vi "Main3.vi"() -> ()   [LabVIEW 2014]
uses:
  TypeDefs/Errors.ctl
  TypeDefs/Data Info.ctl
  <vilib>/Utility/file.llb/Read From Spreadsheet File (string).vi
panel:
  out "Cluster 2":T2
  out "Day":T2={"Info 1"={"Last time in range?"=TRUE, "Date"="", "Start index"=0}, "Info 2"={"Last time in range?"=TRUE, "Date"="", "Start index"=0}, "Info 3"={"Last time in range?"=TRUE, "Date"="", "Start index"=0}, "Info 4"={"Last time in range?"=TRUE, "Date"="", "Start index"=0}, "info 5"={"Last time in range?"=TRUE, "Date"="", "Start index"=0}, "Info 6"={"Last time in range?"=TRUE, "Date"="", "Start index"=0}, "Info 7"={"Last time in range?"=TRUE, "Date"="", "Start index"=0}, "Info 8"={"Last time in range?"=TRUE, "Date"="", "Start index"=0}, "Info 9"={"Last time in range?"=TRUE, "Date"="", "Start index"=0}, "Info 10"={"Last time in range?"=TRUE, "Date"="", "Start index"=0}}
  in  "Cluster":T2
  out "Iteration":i32
  out "ADC Count":dbl[](array[numeric])
  out "# of rows":i32
  in  "Tab Control":T3(tab)
  out "Current (mA)":cluster{dbl[], dbl[]}(graph)
  out "XY Graph 10":cluster{dbl[], dbl[]}[](graph)
  out "Digital signals":cluster{dbl[], dbl[]}[](graph)
  out "Errors 1":T4
  out "Current (mA) 2":cluster{dbl[], dbl[]}(graph)
  out "XY Graph 11":cluster{dbl[], dbl[]}[](graph)
  out "Digital signals 3":cluster{dbl[], dbl[]}[](graph)
  out "Errors 2":T4
  out "Digital signals 2":cluster{dbl[], dbl[]}[](graph)
  out "Current (mA) 3":cluster{dbl[], dbl[]}(graph)
  out "XY Graph 12":cluster{dbl[], dbl[]}[](graph)
  out "Errors 3":T4
  out "Digital signals 4":cluster{dbl[], dbl[]}[](graph)
  out "Current (mA) 4":cluster{dbl[], dbl[]}(graph)
  out "XY Graph 13":cluster{dbl[], dbl[]}[](graph)
  out "Errors 11":T4
  out "Digital signals 5":cluster{dbl[], dbl[]}[](graph)
  out "Current (mA) 5":cluster{dbl[], dbl[]}(graph)
  out "XY Graph 14":cluster{dbl[], dbl[]}[](graph)
  out "Errors 4":T4
  out "Digital signals 6":cluster{dbl[], dbl[]}[](graph)
  out "Current (mA) 6":cluster{dbl[], dbl[]}(graph)
  out "XY Graph 15":cluster{dbl[], dbl[]}[](graph)
  out "Errors 5":T4
  out "Digital signals 7":cluster{dbl[], dbl[]}[](graph)
  out "Current (mA) 7":cluster{dbl[], dbl[]}(graph)
  out "XY Graph 16":cluster{dbl[], dbl[]}[](graph)
  out "Errors 6":T4
  out "Digital signals 8":cluster{dbl[], dbl[]}[](graph)
  out "Current (mA) 8":cluster{dbl[], dbl[]}(graph)
  out "XY Graph 17":cluster{dbl[], dbl[]}[](graph)
  out "Errors 7":T4
  out "Digital signals 9":cluster{dbl[], dbl[]}[](graph)
  out "Current (mA) 9":cluster{dbl[], dbl[]}(graph)
  out "XY Graph 18":cluster{dbl[], dbl[]}[](graph)
  out "Errors 8":T4
  out "Digital signals 10":cluster{dbl[], dbl[]}[](graph)
  out "Current (mA) 10":cluster{dbl[], dbl[]}(graph)
  out "XY Graph 19":cluster{dbl[], dbl[]}[](graph)
  out "Errors 9":T4
  out "subarray":string[][](array[string])
  out "subarray 3":string[](array[string])
  in  "stop":bool
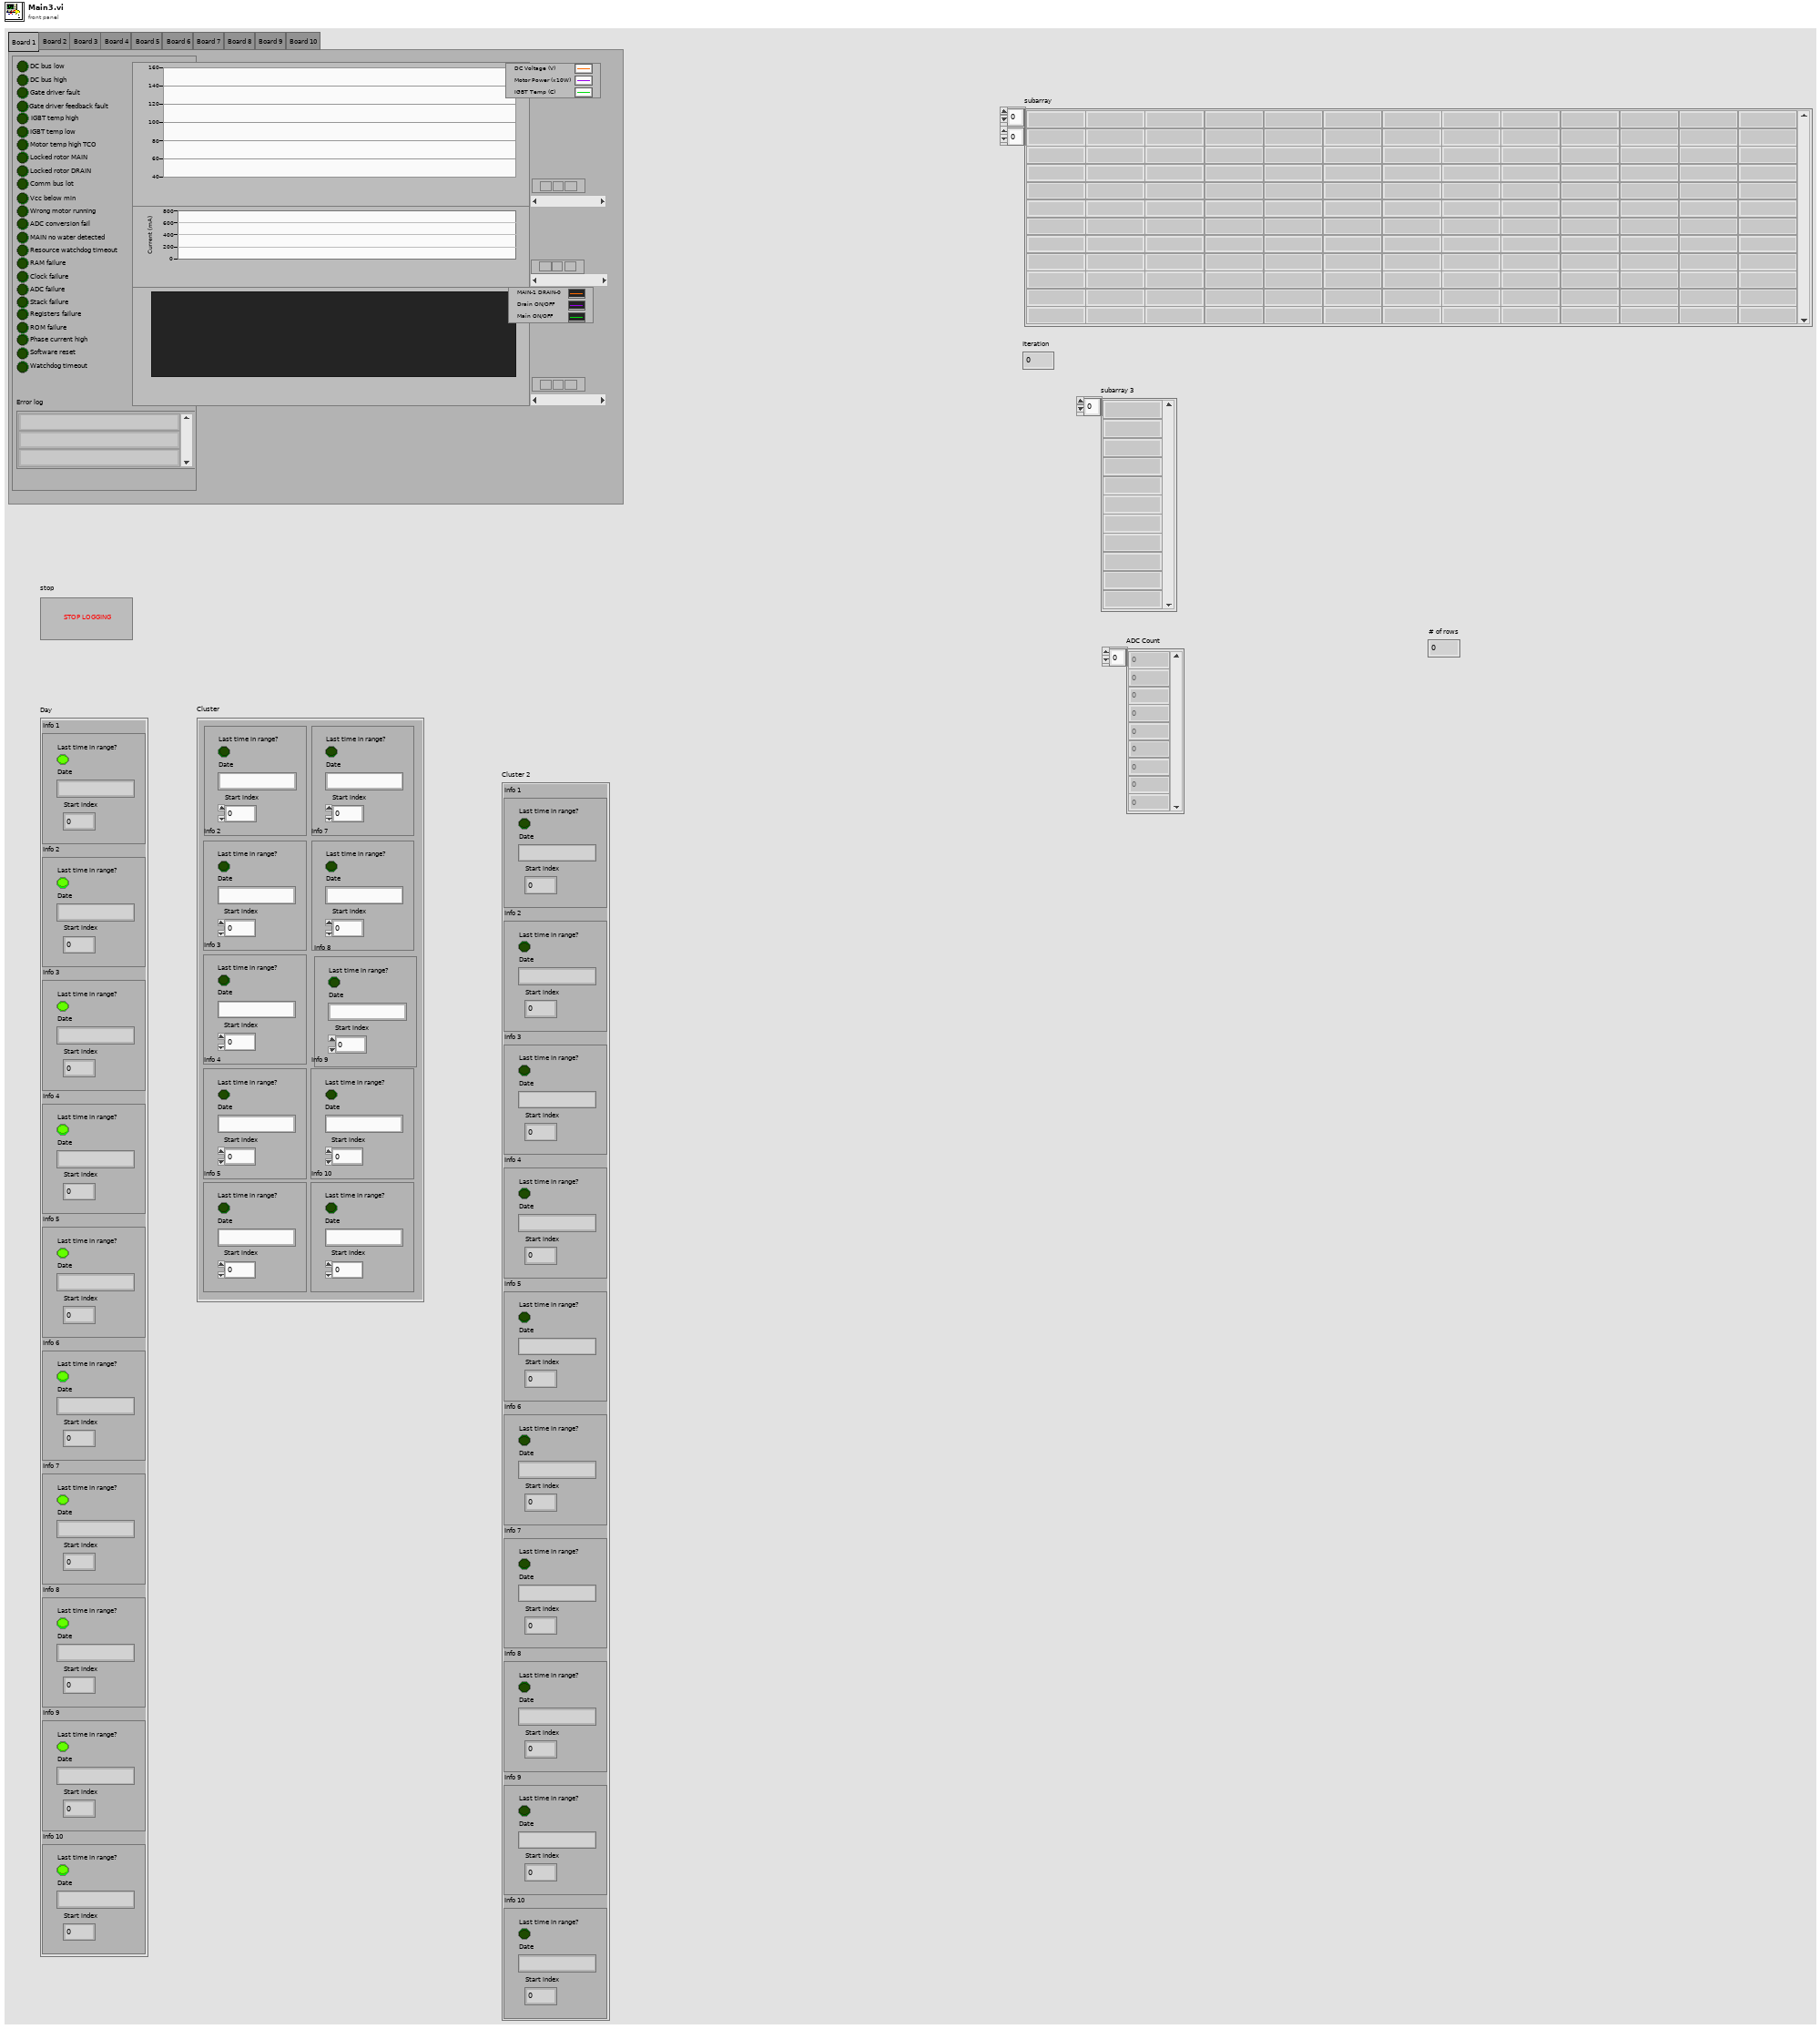
[diagram p1: front panel]
types:
  T1 = typedef "Data Info.ctl" = cluster{"Last time in range?":bool, "Date":string, "Start index":i32}
  T2 = cluster{"Info 1":T1, "Info 2":T1, "Info 3":T1, "Info 4":T1, "info 5":T1, "Info 6":T1, "Info 7":T1, "Info 8":T1, "Info 9":T1, "Info 10":T1}
  T3 = enum32{"Board 1", "Board 2", "Board 3", "Board 4", "Board 5", "Board 6", "Board 7", "Board 8", "Board 9", "Board 10"}
  T4 = typedef "Errors.ctl" = cluster{"DC bus low":bool, "DC bus high":bool, "Gate driver fault":bool, "Gate driver feedback fault":bool, "IGBT temp high":bool, "IGBT temp low":bool, "Motor temp high TCO":bool, "Locked rotor MAIN":bool, "Locked rotor DRAIN":bool, "Comm bus lot":bool, "Vcc below min":bool, "Wrong motor running":bool, "ADC conversion fail":bool, "MAIN no water detected":bool, "Resource watchdog timeout":bool, "RAM failure":bool, "Clock failure":bool, "ADC failure":bool, "Stack failure":bool, "Registers failure":bool, "ROM failure":bool, "Phase current high":bool, "Software reset":bool, "Watchdog timeout":bool, "Error log":string[]}
  T5 = cluster{"01 File Path":path, "02 File Path":path, "03 File Path":path, "04 File Path":path, "05 File Path":path, "06 File Path":path, "07 File Path":path, "08 File Path":path, "09 File Path":path, "10 File Path":path}
  T6 = cluster{"Last time in range?":bool, "date/time string":string, "Start index":i32}
  T7 = cluster{"DC Bus Voltage":dbl, "Current RMS":dbl, "Motor Power":dbl, "IGBT Temp":u16, "Motor Type":u16, "Motor Power Sign":string, "Relay Position":u16, "ADC Count":dbl, "Recirculation Motor ON/OFF":u16, "Drain Motor ON/OFF":u16}
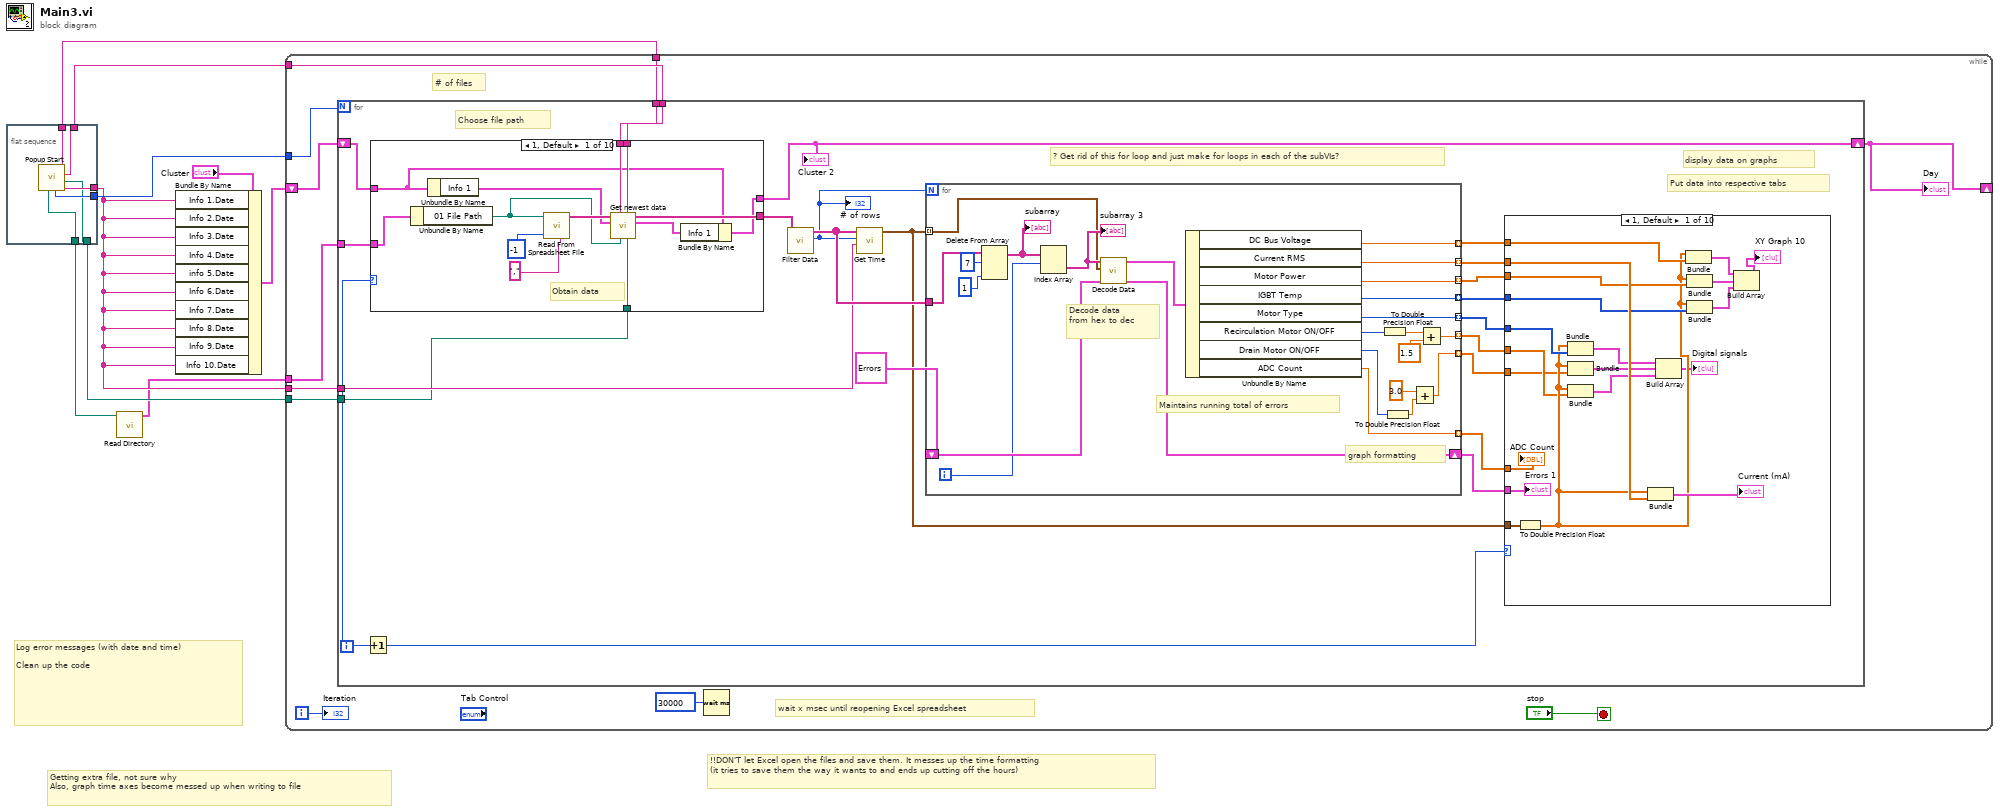
[diagram p0: block diagram]
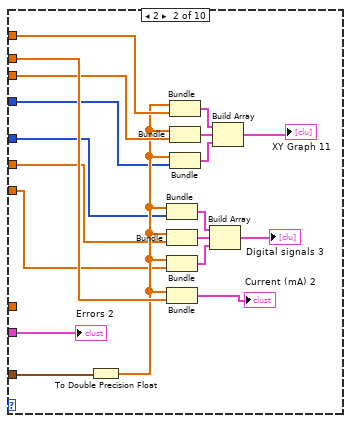
[diagram p2: hidden frame]
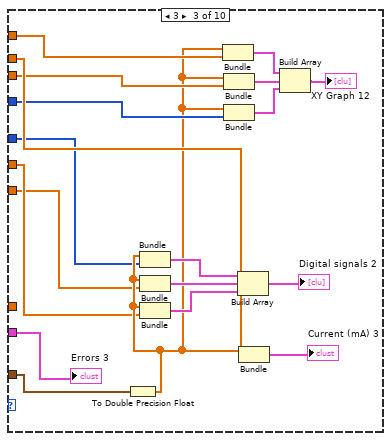
[diagram p3: hidden frame]
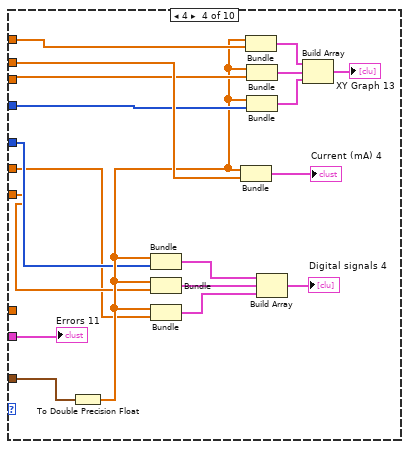
[diagram p4: hidden frame]
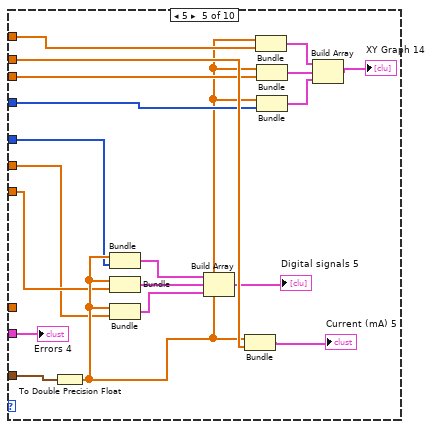
[diagram p5: hidden frame]
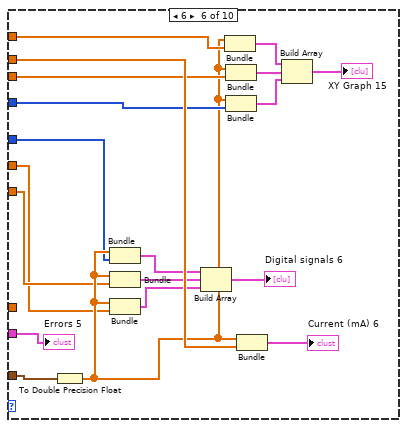
[diagram p6: hidden frame]
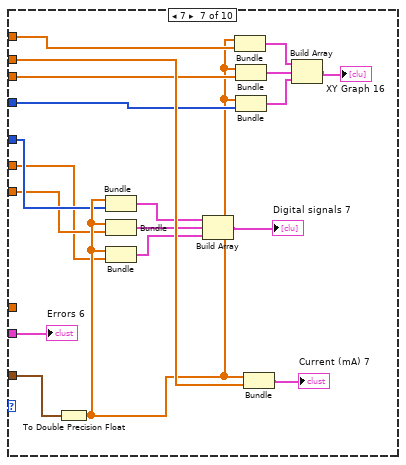
[diagram p7: hidden frame]
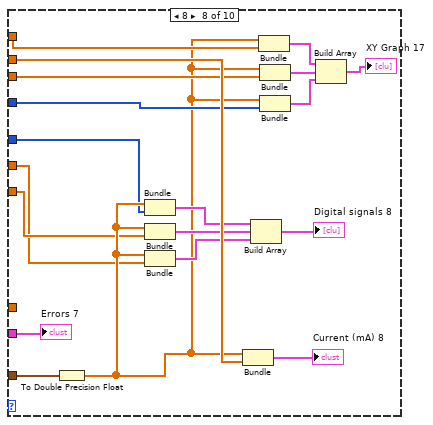
[diagram p8: hidden frame]
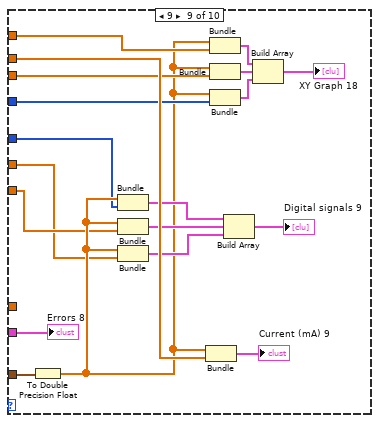
[diagram p9: hidden frame]
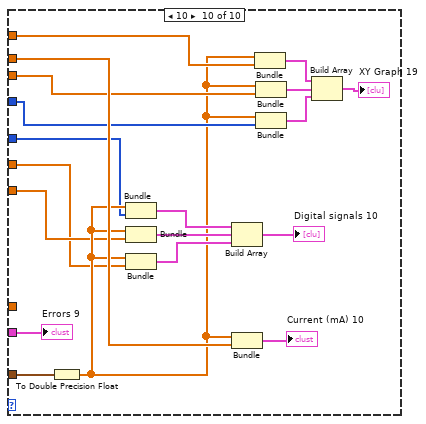
[diagram p10: hidden frame]
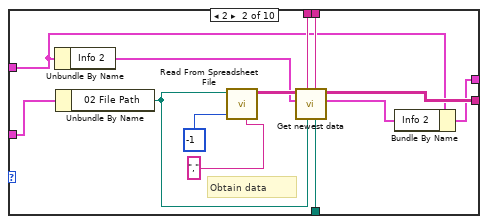
[diagram p11: hidden frame]
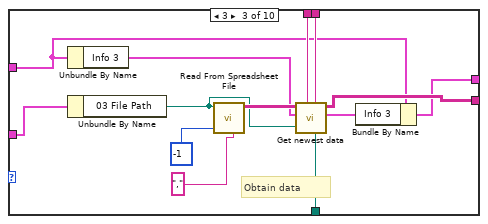
[diagram p12: hidden frame]
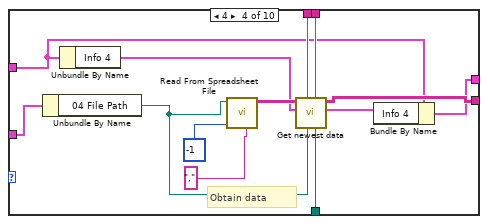
[diagram p13: hidden frame]
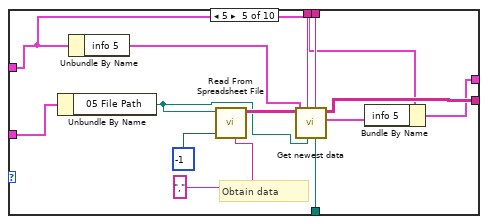
[diagram p14: hidden frame]
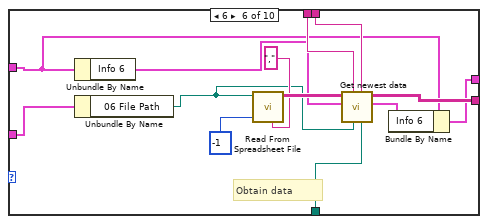
[diagram p15: hidden frame]
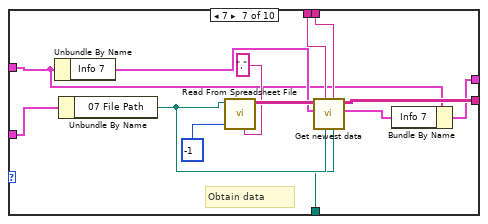
[diagram p16: hidden frame]
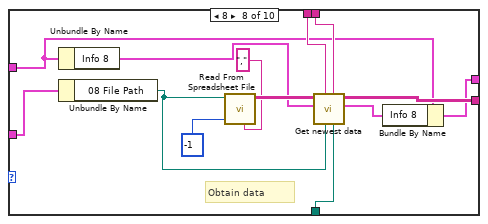
[diagram p17: hidden frame]
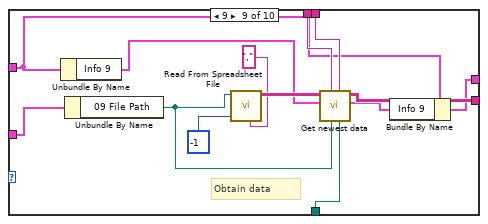
[diagram p18: hidden frame]
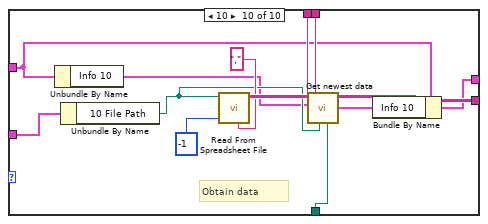
[diagram p19: hidden frame]
diagram:
  # "Getting extra file, not sure why\nAlso, graph time axes become messed up when writing to file"
  # "Log error messages (with date and time)\n\nClean up the code"
  # "!!DON'T let Excel open the files and save them. It messes up the time formatting \n(it tries to save them the way it wants to and ends up cutting off the hours)"
  n1 = flat-sequence {
    tunnel: [w15] -> w3
    tunnel: [w14] -> w7
    tunnel: [w13] -> w1
    tunnel: [w12] -> w6
    tunnel: [w11] -> w5
    tunnel: [w10] -> w4
    frame #0 {
      n2 = call "Popup Start.vi"() -> ("Date Laundry.NET\nstarted (MM_DD) 2"=w15:string, "Folder to store data sets 2"=w12:path, "End time save 2"=w11:string, "Start time save 2"=w10:string, "# of Files 2"=w14:i32, "File directory 2"=w13:path)  [unwired: 6 in]
    }
  }
  n3 = call "Read Directory.vi"("path"=w1) -> ("Laundry.NET \nfile paths 3"=w2:T5)  [unwired: 10 in]
  n4 = Bundle By Name(cluster="Cluster", "Info 1.Date"=w3, "Info 2.Date"=w3, "Info 3.Date"=w3, "Info 4.Date"=w3, "info 5.Date"=w3, "Info 6.Date"=w3, "Info 7.Date"=w3, "Info 8.Date"=w3, "Info 9.Date"=w3, "Info 10.Date"=w3) -> (w8:T2)
  n5 = while {
    shift-right: [w23] -> _
    shift-left: w8 -> [w16]
    tunnel: w3 -> [w22]
    tunnel: w7 -> [w21]
    tunnel: w2 -> [w20]
    tunnel: w6 -> [w19]
    tunnel: w5 -> [w18]
    tunnel: w4 -> [w17]
    i -> [w24]
    stop <- "stop" stop-if-true
    # "# of files"
    # "wait x msec until reopening Excel spreadsheet"
    n6 = for {
      N: w21 -> [_]
      tunnel: w20 -> [w49]
      tunnel: w18 -> [w34]
      tunnel: w22 -> [w32]
      tunnel: w19 -> [w31]
      tunnel: w17 -> [w30]
      shift-right: [w33] -> w23
      shift-left: w16 -> [w27]
      i -> [w48]
      # "? Get rid of this for loop and just make for loops in each of the subVIs?"
      # "display data on graphs"
      # "Put data into respective tabs"
      # "Choose file path"
      n7 = Increment(x=w48) -> (x+1=w47:i32)
      n8 = case shown="1, Default" w47 {
        tunnel: w49 -> [w253 w266 w279 w292 w305 w318 w331 w344 w357 w370]
        tunnel: [w249 w262 w275 w288 w301 w314 w327 w340 w353 w366] -> w35
        tunnel: w31 -> [w247 w258 w271 w284 w297 w312 w323 w336 w349 w362]
        tunnel: w30 -> [w246 w261 w274 w287 w300 w311 w326 w339 w352 w365]
        tunnel: w34 -> [w245 w260 w273 w286 w299 w310 w325 w338 w351 w364]
        tunnel: w27 -> [w242 w255 w269 w281 w294 w307 w320 w333 w346 w360]
        tunnel: [w241 w254 w267 w280 w293 w306 w319 w332 w345 w358] -> w33
        frame 1, Default {
          # "Obtain data"
          n9 = Unbundle By Name(w253) -> ("01 File Path"=w248:path)
          n10 = Unbundle By Name(w242) -> ("Info 1"=w244:T1)
          n11 = call-poly <vilib>:"Read From Spreadsheet File.vi"("delimiter (\\t)"="," ("delimiter (\\t)"), "number of rows (all:-1)"=-1, "file path (dialog if empty)"=w248) -> ("all rows"=w252:string[][])  [unwired: 4 in, 4 out]
          n12 = call "Get newest data.vi"("target path"=w247, "End time"=w245, "source path"=w248, "Start time"=w246, "Previous info"=w244, "all rows"=w252) -> ("New Info"=w243:T6, "newest rows"=w249:string[][])  [unwired: 4 in]
          n13 = Bundle By Name(cluster=w242, "Info 1"=w243) -> (w241:T2)
        }
        frame 2 {
          # "Obtain data"
          n14 = Unbundle By Name(w255) -> ("Info 2"=w257:T1)
          n15 = Unbundle By Name(w266) -> ("02 File Path"=w259:path)
          n16 = call-poly <vilib>:"Read From Spreadsheet File.vi"("delimiter (\\t)"="," ("delimiter (\\t)"), "number of rows (all:-1)"=-1, "file path (dialog if empty)"=w259) -> ("all rows"=w265:string[][])  [unwired: 4 in, 4 out]
          n17 = call "Get newest data.vi"("target path"=w258, "End time"=w260, "source path"=w259, "Start time"=w261, "Previous info"=w257, "all rows"=w265) -> ("New Info"=w256:T6, "newest rows"=w262:string[][])  [unwired: 4 in]
          n18 = Bundle By Name(cluster=w255, "Info 2"=w256) -> (w254:T2)
        }
        frame 3 {
          # "Obtain data"
          n19 = Unbundle By Name(w269) -> ("Info 3"=w270:T1)
          n20 = Unbundle By Name(w279) -> ("03 File Path"=w272:path)
          n21 = call-poly <vilib>:"Read From Spreadsheet File.vi"("delimiter (\\t)"="," ("delimiter (\\t)"), "number of rows (all:-1)"=-1, "file path (dialog if empty)"=w272) -> ("all rows"=w278:string[][])  [unwired: 4 in, 4 out]
          n22 = call "Get newest data.vi"("target path"=w271, "End time"=w273, "source path"=w272, "Start time"=w274, "Previous info"=w270, "all rows"=w278) -> ("New Info"=w268:T6, "newest rows"=w275:string[][])  [unwired: 4 in]
          n23 = Bundle By Name(cluster=w269, "Info 3"=w268) -> (w267:T2)
        }
        frame 4 {
          # "Obtain data"
          n24 = Unbundle By Name(w292) -> ("04 File Path"=w285:path)
          n25 = Unbundle By Name(w281) -> ("Info 4"=w283:T1)
          n26 = call-poly <vilib>:"Read From Spreadsheet File.vi"("delimiter (\\t)"="," ("delimiter (\\t)"), "number of rows (all:-1)"=-1, "file path (dialog if empty)"=w285) -> ("all rows"=w291:string[][])  [unwired: 4 in, 4 out]
          n27 = call "Get newest data.vi"("target path"=w284, "End time"=w286, "source path"=w285, "Start time"=w287, "Previous info"=w283, "all rows"=w291) -> ("New Info"=w282:T6, "newest rows"=w288:string[][])  [unwired: 4 in]
          n28 = Bundle By Name(cluster=w281, "Info 4"=w282) -> (w280:T2)
        }
        frame 5 {
          # "Obtain data"
          n29 = Unbundle By Name(w305) -> ("05 File Path"=w298:path)
          n30 = Unbundle By Name(w294) -> ("info 5"=w296:T1)
          n31 = call-poly <vilib>:"Read From Spreadsheet File.vi"("delimiter (\\t)"="," ("delimiter (\\t)"), "number of rows (all:-1)"=-1, "file path (dialog if empty)"=w298) -> ("all rows"=w304:string[][])  [unwired: 4 in, 4 out]
          n32 = call "Get newest data.vi"("target path"=w297, "End time"=w299, "source path"=w298, "Start time"=w300, "Previous info"=w296, "all rows"=w304) -> ("New Info"=w295:T6, "newest rows"=w301:string[][])  [unwired: 4 in]
          n33 = Bundle By Name(cluster=w294, "info 5"=w295) -> (w293:T2)
        }
        frame 6 {
          # "Obtain data"
          n34 = Unbundle By Name(w307) -> ("Info 6"=w309:T1)
          n35 = Unbundle By Name(w318) -> ("06 File Path"=w313:path)
          n36 = call-poly <vilib>:"Read From Spreadsheet File.vi"("delimiter (\\t)"="," ("delimiter (\\t)"), "number of rows (all:-1)"=-1, "file path (dialog if empty)"=w313) -> ("all rows"=w317:string[][])  [unwired: 4 in, 4 out]
          n37 = call "Get newest data.vi"("target path"=w312, "End time"=w310, "source path"=w313, "Start time"=w311, "Previous info"=w309, "all rows"=w317) -> ("New Info"=w308:T6, "newest rows"=w314:string[][])  [unwired: 4 in]
          n38 = Bundle By Name(cluster=w307, "Info 6"=w308) -> (w306:T2)
        }
        frame 7 {
          # "Obtain data"
          n39 = Unbundle By Name(w320) -> ("Info 7"=w322:T1)
          n40 = Unbundle By Name(w331) -> ("07 File Path"=w324:path)
          n41 = call-poly <vilib>:"Read From Spreadsheet File.vi"("delimiter (\\t)"="," ("delimiter (\\t)"), "number of rows (all:-1)"=-1, "file path (dialog if empty)"=w324) -> ("all rows"=w330:string[][])  [unwired: 4 in, 4 out]
          n42 = call "Get newest data.vi"("target path"=w323, "End time"=w325, "source path"=w324, "Start time"=w326, "Previous info"=w322, "all rows"=w330) -> ("New Info"=w321:T6, "newest rows"=w327:string[][])  [unwired: 4 in]
          n43 = Bundle By Name(cluster=w320, "Info 7"=w321) -> (w319:T2)
        }
        frame 8 {
          # "Obtain data"
          n44 = Unbundle By Name(w333) -> ("Info 8"=w335:T1)
          n45 = Unbundle By Name(w344) -> ("08 File Path"=w337:path)
          n46 = call-poly <vilib>:"Read From Spreadsheet File.vi"("delimiter (\\t)"="," ("delimiter (\\t)"), "number of rows (all:-1)"=-1, "file path (dialog if empty)"=w337) -> ("all rows"=w343:string[][])  [unwired: 4 in, 4 out]
          n47 = call "Get newest data.vi"("target path"=w336, "End time"=w338, "source path"=w337, "Start time"=w339, "Previous info"=w335, "all rows"=w343) -> ("New Info"=w334:T6, "newest rows"=w340:string[][])  [unwired: 4 in]
          n48 = Bundle By Name(cluster=w333, "Info 8"=w334) -> (w332:T2)
        }
        frame 9 {
          # "Obtain data"
          n49 = Unbundle By Name(w346) -> ("Info 9"=w348:T1)
          n50 = Unbundle By Name(w357) -> ("09 File Path"=w350:path)
          n51 = call-poly <vilib>:"Read From Spreadsheet File.vi"("delimiter (\\t)"="," ("delimiter (\\t)"), "number of rows (all:-1)"=-1, "file path (dialog if empty)"=w350) -> ("all rows"=w356:string[][])  [unwired: 4 in, 4 out]
          n52 = call "Get newest data.vi"("target path"=w349, "End time"=w351, "source path"=w350, "Start time"=w352, "Previous info"=w348, "all rows"=w356) -> ("New Info"=w347:T6, "newest rows"=w353:string[][])  [unwired: 4 in]
          n53 = Bundle By Name(cluster=w346, "Info 9"=w347) -> (w345:T2)
        }
        frame 10 {
          # "Obtain data"
          n54 = Unbundle By Name(w360) -> ("Info 10"=w361:T1)
          n55 = Unbundle By Name(w370) -> ("10 File Path"=w363:path)
          n56 = call-poly <vilib>:"Read From Spreadsheet File.vi"("delimiter (\\t)"="," ("delimiter (\\t)"), "number of rows (all:-1)"=-1, "file path (dialog if empty)"=w363) -> ("all rows"=w369:string[][])  [unwired: 4 in, 4 out]
          n57 = call "Get newest data.vi"("target path"=w362, "End time"=w364, "source path"=w363, "Start time"=w365, "Previous info"=w361, "all rows"=w369) -> ("New Info"=w359:T6, "newest rows"=w366:string[][])  [unwired: 4 in]
          n58 = Bundle By Name(cluster=w360, "Info 10"=w359) -> (w358:T2)
        }
      }
      "Cluster 2" <- w33
      n59 = call "Filter Data.vi"("All Rows"=w35) -> ("element"=w28:i32, "new array"=w40:string[][])  [unwired: 9 in]
      "# of rows" <- w28
      n60 = call "Get Time.vi"("Date"=w32, "# of rows"=w28, "Data row"=w40) -> ("Time array"=w29:timestamp[])  [unwired: 8 in]
      n61 = for {
        N: w28 -> [_]
        tunnel: [w394] -> w44 mode=indexing
        tunnel: [w393] -> w46 mode=indexing
        tunnel: [w392] -> w45 mode=indexing
        tunnel: [w391] -> w43 mode=indexing
        tunnel: [w390] -> w42 mode=indexing
        shift-right: [w377] -> w41
        shift-left: T4 {"DC bus low"=FALSE, "DC bus high"=FALSE, "Gate driver fault"=FALSE, "Gate driver feedback fault"=FALSE, "IGBT temp high"=FALSE, "IGBT temp low"=FALSE, "Motor temp high TCO"=FALSE, "Locked rotor MAIN"=FALSE, "Locked rotor DRAIN"=FALSE, "Comm bus lot"=FALSE, "Vcc below min"=FALSE, "Wrong motor running"=FALSE, "ADC conversion fail"=FALSE, "MAIN no water detected"=FALSE, "Resource watchdog timeout"=FALSE, "RAM failure"=FALSE, "Clock failure"=FALSE, "ADC failure"=FALSE, "Stack failure"=FALSE, "Registers failure"=FALSE, "ROM failure"=FALSE, "Phase current high"=FALSE, "Software reset"=FALSE, "Watchdog timeout"=FALSE, "Error log"=[]} ("Errors Out") -> [w389]
        tunnel: w40 -> [w376]
        tunnel: [w386] -> w37 mode=indexing
        tunnel: [w385] -> w38 mode=indexing
        tunnel: [w378] -> w36 mode=indexing
        tunnel: w29 -> [w371] mode=indexing
        i -> [w372]
        # "graph formatting"
        # "Maintains running total of errors"
        # "Decode data\nfrom hex to dec"
        n62 = Delete From Array(array=w376, length=7, index (col)=1 ("disabled index (col)")) -> (array with subset deleted=w373:string[][])  [unwired: 1 in, 1 out]
        "subarray" <- w373
        n63 = Index Array(array=w373, index (row)=w372) -> (element=w387:string[])  [unwired: 1 in]
        "subarray 3" <- w387
        n64 = call "Decode Data.vi"("Errors In"=w389, "Time Stamp"=w371, "Data Array"=w387) -> ("Errors Out"=w377:T4, "logData Out"=w388:T7)  [unwired: 7 in]
        n65 = Unbundle By Name(w388) -> ("DC Bus Voltage"=w394:dbl, "Current RMS"=w393:dbl, "Motor Power"=w392:dbl, "IGBT Temp"=w391:u16, "Motor Type"=w390:u16, "Recirculation Motor ON/OFF"=w384:u16, "Drain Motor ON/OFF"=w381:u16, "ADC Count"=w378:dbl)
        n66 = To Double Precision Float(number=w384) -> (double precision float=w383:dbl)
        n67 = To Double Precision Float(number=w381) -> (double precision float=w380:dbl)
        n68 = Add(x=3.0, y=w380) -> (x+y=w385:dbl)
        n69 = Add(x=w383, y=1.5) -> (x+y=w386:dbl)
      }
      n70 = case shown="1, Default" w47 {
        tunnel: w46 -> [w68 w87 w106 w125 w144 w163 w182 w201 w220 w239]
        tunnel: w45 -> [w60 w82 w101 w119 w139 w158 w177 w196 w216 w237]
        tunnel: w44 -> [w61 w83 w102 w121 w140 w159 w178 w197 w217 w238]
        tunnel: w43 -> [w59 w77 w100 w120 w138 w157 w176 w195 w215 w236]
        tunnel: w42 -> [w58 w70 w95 w114 w133 w152 w171 w190 w209 w228]
        tunnel: w41 -> [w69 w73 w89 w110 w130 w148 w168 w187 w206 w224]
        tunnel: w29 -> [w67 w88 w107 w126 w145 w164 w183 w202 w221 w240]
        tunnel: w37 -> [w56 w76 w94 w112 w131 w150 w169 w188 w207 w226]
        tunnel: w38 -> [w55 w75 w93 w113 w132 w151 w170 w189 w208 w227]
        tunnel: w36 -> [w50 _ _ _ _ _ _ _ _ _]
        frame 1, Default {
          n71 = To Double Precision Float(number=w67) -> (double precision float=w57:dbl[])
          n72 = Bundle(w57, w58) -> (w54:cluster{dbl[], u16[]})  [unwired: 1 in]
          n73 = Bundle(w57, w55) -> (w52:cluster{dbl[], dbl[]})  [unwired: 1 in]
          n74 = Bundle(w57, w56) -> (w51:cluster{dbl[], dbl[]})  [unwired: 1 in]
          n75 = Bundle(w57, w68) -> (→"Current (mA)":cluster{dbl[], dbl[]})  [unwired: 1 in]
          n76 = Build Array(w54, w52, w51) -> (→"Digital signals":cluster{dbl[], dbl[]}[])
          n77 = Bundle(w57, w61) -> (w65:cluster{dbl[], dbl[]})  [unwired: 1 in]
          n78 = Bundle(w57, w60) -> (w64:cluster{dbl[], dbl[]})  [unwired: 1 in]
          n79 = Bundle(w57, w59) -> (w63:cluster{dbl[], u16[]})  [unwired: 1 in]
          n80 = Build Array(w65, w64, w63) -> (→"XY Graph 10":cluster{dbl[], dbl[]}[])
          "Errors 1" <- w69
          "ADC Count" <- w50
        }
        frame 2 {
          n81 = To Double Precision Float(number=w88) -> (double precision float=w78:dbl[])
          n82 = Bundle(w78, w70) -> (w81:cluster{dbl[], u16[]})  [unwired: 1 in]
          n83 = Bundle(w78, w76) -> (w80:cluster{dbl[], dbl[]})  [unwired: 1 in]
          n84 = Bundle(w78, w75) -> (w79:cluster{dbl[], dbl[]})  [unwired: 1 in]
          n85 = Bundle(w78, w87) -> (→"Current (mA) 2":cluster{dbl[], dbl[]})  [unwired: 1 in]
          n86 = Bundle(w78, w83) -> (w86:cluster{dbl[], dbl[]})  [unwired: 1 in]
          n87 = Bundle(w78, w82) -> (w85:cluster{dbl[], dbl[]})  [unwired: 1 in]
          n88 = Bundle(w78, w77) -> (w84:cluster{dbl[], u16[]})  [unwired: 1 in]
          n89 = Build Array(w81, w80, w79) -> (→"Digital signals 3":cluster{dbl[], dbl[]}[])
          n90 = Build Array(w86, w85, w84) -> (→"XY Graph 11":cluster{dbl[], dbl[]}[])
          "Errors 2" <- w73
        }
        frame 3 {
          n91 = To Double Precision Float(number=w107) -> (double precision float=w96:dbl[])
          n92 = Bundle(w96, w95) -> (w99:cluster{dbl[], u16[]})  [unwired: 1 in]
          n93 = Bundle(w96, w93) -> (w98:cluster{dbl[], dbl[]})  [unwired: 1 in]
          n94 = Bundle(w96, w94) -> (w97:cluster{dbl[], dbl[]})  [unwired: 1 in]
          n95 = Bundle(w96, w102) -> (w105:cluster{dbl[], dbl[]})  [unwired: 1 in]
          n96 = Bundle(w96, w101) -> (w104:cluster{dbl[], dbl[]})  [unwired: 1 in]
          n97 = Bundle(w96, w100) -> (w103:cluster{dbl[], u16[]})  [unwired: 1 in]
          n98 = Build Array(w99, w98, w97) -> (→"Digital signals 2":cluster{dbl[], dbl[]}[])
          n99 = Bundle(w96, w106) -> (→"Current (mA) 3":cluster{dbl[], dbl[]})  [unwired: 1 in]
          n100 = Build Array(w105, w104, w103) -> (→"XY Graph 12":cluster{dbl[], dbl[]}[])
          "Errors 3" <- w89
        }
        frame 4 {
          n101 = To Double Precision Float(number=w126) -> (double precision float=w115:dbl[])
          n102 = Bundle(w115, w114) -> (w118:cluster{dbl[], u16[]})  [unwired: 1 in]
          n103 = Bundle(w115, w113) -> (w117:cluster{dbl[], dbl[]})  [unwired: 1 in]
          n104 = Bundle(w115, w112) -> (w116:cluster{dbl[], dbl[]})  [unwired: 1 in]
          n105 = Bundle(w115, w125) -> (→"Current (mA) 4":cluster{dbl[], dbl[]})  [unwired: 1 in]
          n106 = Bundle(w115, w121) -> (w124:cluster{dbl[], dbl[]})  [unwired: 1 in]
          n107 = Bundle(w115, w119) -> (w123:cluster{dbl[], dbl[]})  [unwired: 1 in]
          n108 = Bundle(w115, w120) -> (w122:cluster{dbl[], u16[]})  [unwired: 1 in]
          n109 = Build Array(w118, w117, w116) -> (→"Digital signals 4":cluster{dbl[], dbl[]}[])
          n110 = Build Array(w124, w123, w122) -> (→"XY Graph 13":cluster{dbl[], dbl[]}[])
          "Errors 11" <- w110
        }
        frame 5 {
          n111 = To Double Precision Float(number=w145) -> (double precision float=w134:dbl[])
          n112 = Bundle(w134, w133) -> (w137:cluster{dbl[], u16[]})  [unwired: 1 in]
          n113 = Bundle(w134, w132) -> (w136:cluster{dbl[], dbl[]})  [unwired: 1 in]
          n114 = Bundle(w134, w131) -> (w135:cluster{dbl[], dbl[]})  [unwired: 1 in]
          n115 = Build Array(w137, w136, w135) -> (→"Digital signals 5":cluster{dbl[], dbl[]}[])
          n116 = Bundle(w134, w144) -> (→"Current (mA) 5":cluster{dbl[], dbl[]})  [unwired: 1 in]
          n117 = Bundle(w134, w140) -> (w143:cluster{dbl[], dbl[]})  [unwired: 1 in]
          n118 = Bundle(w134, w139) -> (w142:cluster{dbl[], dbl[]})  [unwired: 1 in]
          n119 = Bundle(w134, w138) -> (w141:cluster{dbl[], u16[]})  [unwired: 1 in]
          n120 = Build Array(w143, w142, w141) -> (→"XY Graph 14":cluster{dbl[], dbl[]}[])
          "Errors 4" <- w130
        }
        frame 6 {
          n121 = To Double Precision Float(number=w164) -> (double precision float=w153:dbl[])
          n122 = Bundle(w153, w152) -> (w156:cluster{dbl[], u16[]})  [unwired: 1 in]
          n123 = Bundle(w153, w151) -> (w155:cluster{dbl[], dbl[]})  [unwired: 1 in]
          n124 = Bundle(w153, w150) -> (w154:cluster{dbl[], dbl[]})  [unwired: 1 in]
          n125 = Build Array(w156, w155, w154) -> (→"Digital signals 6":cluster{dbl[], dbl[]}[])
          n126 = Bundle(w153, w159) -> (w162:cluster{dbl[], dbl[]})  [unwired: 1 in]
          n127 = Bundle(w153, w158) -> (w161:cluster{dbl[], dbl[]})  [unwired: 1 in]
          n128 = Bundle(w153, w157) -> (w160:cluster{dbl[], u16[]})  [unwired: 1 in]
          n129 = Bundle(w153, w163) -> (→"Current (mA) 6":cluster{dbl[], dbl[]})  [unwired: 1 in]
          n130 = Build Array(w162, w161, w160) -> (→"XY Graph 15":cluster{dbl[], dbl[]}[])
          "Errors 5" <- w148
        }
        frame 7 {
          n131 = To Double Precision Float(number=w183) -> (double precision float=w172:dbl[])
          n132 = Bundle(w172, w171) -> (w175:cluster{dbl[], u16[]})  [unwired: 1 in]
          n133 = Bundle(w172, w170) -> (w174:cluster{dbl[], dbl[]})  [unwired: 1 in]
          n134 = Bundle(w172, w169) -> (w173:cluster{dbl[], dbl[]})  [unwired: 1 in]
          n135 = Build Array(w175, w174, w173) -> (→"Digital signals 7":cluster{dbl[], dbl[]}[])
          n136 = Bundle(w172, w178) -> (w181:cluster{dbl[], dbl[]})  [unwired: 1 in]
          n137 = Bundle(w172, w177) -> (w180:cluster{dbl[], dbl[]})  [unwired: 1 in]
          n138 = Bundle(w172, w176) -> (w179:cluster{dbl[], u16[]})  [unwired: 1 in]
          n139 = Bundle(w172, w182) -> (→"Current (mA) 7":cluster{dbl[], dbl[]})  [unwired: 1 in]
          n140 = Build Array(w181, w180, w179) -> (→"XY Graph 16":cluster{dbl[], dbl[]}[])
          "Errors 6" <- w168
        }
        frame 8 {
          n141 = To Double Precision Float(number=w202) -> (double precision float=w191:dbl[])
          n142 = Bundle(w191, w190) -> (w194:cluster{dbl[], u16[]})  [unwired: 1 in]
          n143 = Bundle(w191, w189) -> (w193:cluster{dbl[], dbl[]})  [unwired: 1 in]
          n144 = Bundle(w191, w188) -> (w192:cluster{dbl[], dbl[]})  [unwired: 1 in]
          n145 = Bundle(w191, w201) -> (→"Current (mA) 8":cluster{dbl[], dbl[]})  [unwired: 1 in]
          n146 = Build Array(w194, w193, w192) -> (→"Digital signals 8":cluster{dbl[], dbl[]}[])
          n147 = Bundle(w191, w197) -> (w200:cluster{dbl[], dbl[]})  [unwired: 1 in]
          n148 = Bundle(w191, w196) -> (w199:cluster{dbl[], dbl[]})  [unwired: 1 in]
          n149 = Bundle(w191, w195) -> (w198:cluster{dbl[], u16[]})  [unwired: 1 in]
          n150 = Build Array(w200, w199, w198) -> (→"XY Graph 17":cluster{dbl[], dbl[]}[])
          "Errors 7" <- w187
        }
        frame 9 {
          n151 = To Double Precision Float(number=w221) -> (double precision float=w210:dbl[])
          n152 = Bundle(w210, w209) -> (w213:cluster{dbl[], u16[]})  [unwired: 1 in]
          n153 = Bundle(w210, w208) -> (w212:cluster{dbl[], dbl[]})  [unwired: 1 in]
          n154 = Bundle(w210, w207) -> (w211:cluster{dbl[], dbl[]})  [unwired: 1 in]
          n155 = Bundle(w210, w220) -> (→"Current (mA) 9":cluster{dbl[], dbl[]})  [unwired: 1 in]
          n156 = Bundle(w210, w217) -> (w219:cluster{dbl[], dbl[]})  [unwired: 1 in]
          n157 = Bundle(w210, w216) -> (w218:cluster{dbl[], dbl[]})  [unwired: 1 in]
          n158 = Bundle(w210, w215) -> (w214:cluster{dbl[], u16[]})  [unwired: 1 in]
          n159 = Build Array(w213, w212, w211) -> (→"Digital signals 9":cluster{dbl[], dbl[]}[])
          n160 = Build Array(w219, w218, w214) -> (→"XY Graph 18":cluster{dbl[], dbl[]}[])
          "Errors 8" <- w206
        }
        frame 10 {
          n161 = To Double Precision Float(number=w240) -> (double precision float=w229:dbl[])
          n162 = Bundle(w229, w228) -> (w232:cluster{dbl[], u16[]})  [unwired: 1 in]
          n163 = Bundle(w229, w227) -> (w231:cluster{dbl[], dbl[]})  [unwired: 1 in]
          n164 = Bundle(w229, w226) -> (w230:cluster{dbl[], dbl[]})  [unwired: 1 in]
          n165 = Build Array(w232, w231, w230) -> (→"Digital signals 10":cluster{dbl[], dbl[]}[])
          n166 = Bundle(w229, w239) -> (→"Current (mA) 10":cluster{dbl[], dbl[]})  [unwired: 1 in]
          n167 = Bundle(w229, w238) -> (w235:cluster{dbl[], dbl[]})  [unwired: 1 in]
          n168 = Bundle(w229, w237) -> (w234:cluster{dbl[], dbl[]})  [unwired: 1 in]
          n169 = Bundle(w229, w236) -> (w233:cluster{dbl[], u16[]})  [unwired: 1 in]
          n170 = Build Array(w235, w234, w233) -> (→"XY Graph 19":cluster{dbl[], dbl[]}[])
          "Errors 9" <- w224
        }
      }
    }
    "Day" <- w23
    n171 = Wait (ms)(milliseconds to wait=u32 30000) -> ()  [unwired: 1 out]
    "Iteration" <- w24
  }
